vi "SCLN_ServerLoop1.vi"(1 "Server Port":i32, 3 "Client Number":i32, 4 "Server Number":i32, 5 "TCP IN":refnum<k5>) -> (0 "Server Out":i32, 2 "TCP OUT":refnum<k5>)   [LabVIEW 2015]
uses:
  SCLN_RW_Select.ctl
panel:
  out "Client IP":string
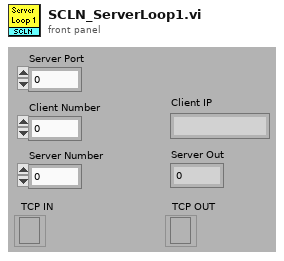
[diagram p1: front panel]
types:
  T1 = typedef "SCLN_RW_Select.ctl" = enum16{"Read", "Write"}
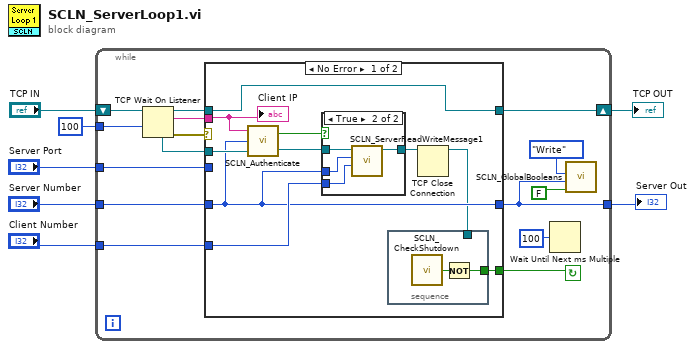
[diagram p0: block diagram]
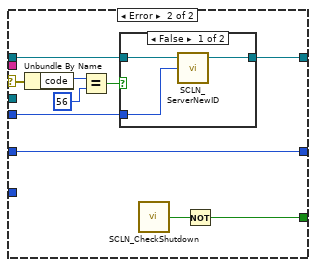
[diagram p3: hidden frame]
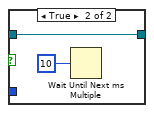
[diagram p4: hidden frame]
diagram:
  n1 = while {
    tunnel: "Server Number" -> [w21]
    tunnel: [w17] -> w5
    tunnel: "Client Number" -> [w15]
    tunnel: "Server Port" -> [w13]
    shift-right: [w11] -> w3
    shift-left: "TCP IN" -> [w10]
    tunnel: 100 -> [w9]
    stop <- w22 continue-if-true
    n2 = TCP Wait On Listener(9:w9, 11:w10) -> (0:w19:errorcluster, 2:w14:string, 3:w12:refnum<k5>, 4:w20:refnum<k5>)  [unwired: 2 in, 1 out]
    n3 = case shown="No Error" w19 {
      selector: w19 -> [_ w46]
      tunnel: [w32 w49] -> w22
      tunnel: w21 -> [w27 w48]
      tunnel: w20 -> [w31 _]
      tunnel: [w27 w48] -> w17
      tunnel: w15 -> [w28 _]
      tunnel: w14 -> [w26 _]
      tunnel: w13 -> [_ w41]
      tunnel: w12 -> [w23 w42]
      tunnel: [w23 w40] -> w11
      frame No Error {
        n4 = call "SCLN_Authenticate.vi"("TCP IN"=w31, "Server Number"=w27, "Computer Name"=w26) -> ("TCP OUT"=w29:refnum<k5>, "Authentic"=w30:bool)
        n5 = case shown="True" w30 {
          tunnel: [w33 w37] -> w25
          tunnel: w29 -> [w33 w36]
          tunnel: w27 -> [_ w35]
          tunnel: w28 -> [_ w34]
          frame False {
          }
          frame True {
            n6 = call "SCLN_ServerReadWriteMessage1.vi"("Client Number"=w34, "Server Number"=w35, "TCP ID In"=w36) -> ("TCP ID Out"=w37:refnum<k5>)  [unwired: 1 in, 1 out]
          }
        }
        n7 = TCP Close Connection(connection ID=w25) -> (connection ID out=w24:refnum<k5>)  [unwired: 2 in, 1 out]
        n8 = stacked-sequence {
          tunnel: [w38] -> w32
          tunnel: w24 -> [_]
          frame #0 {
            n9 = call "SCLN_CheckShutdown.vi"() -> ("Shutdown"=w39:bool)
            n10 = Not(x=w39) -> (.not. x?=w38:bool)
          }
        }
        "Client IP" <- w26
      }
      frame Error {
        n11 = Unbundle By Name(w46) -> ("code"=w45:i32)
        n12 = Equal?(x=w45, y=56) -> (x = y?=w43:bool)
        n13 = case shown="False" w43 {
          tunnel: w42 -> [w50 w53]
          tunnel: w41 -> [w52 _]
          tunnel: [w51 w53] -> w40
          frame False {
            n14 = call "SCLN_ServerNewID.vi"("Server Port"=w52, "Listener ID IN"=w50) -> ("Listener ID OUT"=w51:refnum<k5>)  [unwired: 2 in]
          }
          frame True {
            n15 = Wait Until Next ms Multiple(millisecond multiple=10) -> ()  [unwired: 1 out]
          }
        }
        n16 = call "SCLN_CheckShutdown.vi"() -> ("Shutdown"=w47:bool)
        n17 = Not(x=w47) -> (.not. x?=w49:bool)
      }
    }
    n18 = Wait Until Next ms Multiple(millisecond multiple=100) -> ()  [unwired: 1 out]
    n19 = call "SCLN_GlobalBooleans.vi"("Write Value"=FALSE, "Element"=w17, "Operation"=SCLN_RW_Select."Write" ("GBL_RW")) -> ()  [unwired: 1 in, 2 out]
  }
  "TCP OUT" <- w3
  "Server Out" <- w5
